vi "Rectangle Comparison.vi"(6 "Line Border":cluster{"Top":dbl, "Bottom":dbl}={"Top"=6.0, "Bottom"=1.0}, 9 "Second":dbl[](array[numeric]), 11 "First":dbl[](array[numeric])) -> (0 "Rect":T1, 1 "Line":T1, 3 "Scores":T2)   [LabVIEW 2016]
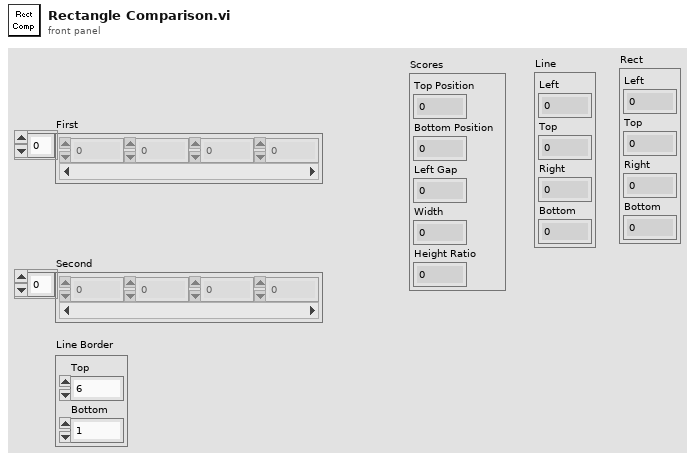
[diagram p1: front panel]
types:
  T1 = cluster{"Left":dbl, "Top":dbl, "Right":dbl, "Bottom":dbl}
  T2 = cluster{"Top Position":dbl, "Bottom Position":dbl, "Left Gap":dbl, "Width":dbl, "Height Ratio":dbl}
  T3 = cluster{"[0]":dbl, "[1]":dbl, "[2]":dbl, "[3]":dbl}
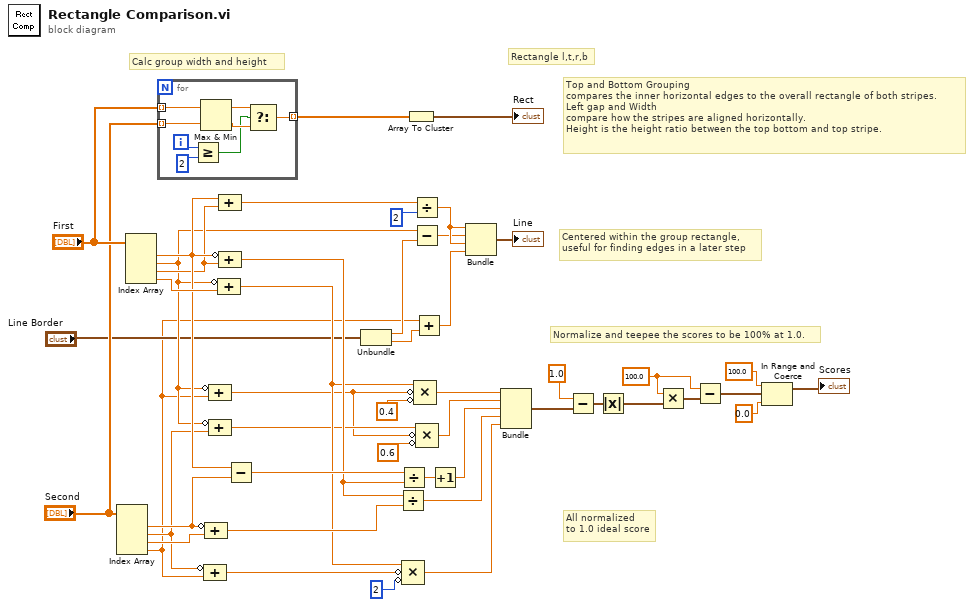
[diagram p0: block diagram]
diagram:
  w20 = 100.0 ("x/y")
  # "Centered within the group rectangle,\nuseful for finding edges in a later step"
  # "All normalized\nto 1.0 ideal score"
  # "Normalize and teepee the scores to be 100% at 1.0."
  # "Top and Bottom Grouping\ncompares the inner horizontal edges to the overall rectangle of both stripes.\nLeft gap and Width\ncompare how the stripes are aligned horizontally.\nHeight is the height ratio between the top bottom and top stripe."
  # "Calc group width and height"
  # "Rectangle l,t,r,b"
  n1 = Index Array(array="Second") -> (element #1=w44:dbl, element #2=w11:dbl, element #3=w47:dbl, element #4=w1:dbl)  [unwired: 4 in]
  n2 = Index Array(array="First") -> (element #1=w36:dbl, element #2=w10:dbl, element #3=w35:dbl, element #4=w37:dbl)  [unwired: 4 in]
  n3 = for {
    tunnel: "First" -> [w55] mode=indexing
    tunnel: "Second" -> [w54] mode=indexing
    tunnel: [w48] -> w27 mode=indexing
    i -> [w52]
    n4 = Greater Or Equal?(x=w52, y=2) -> (x >= y?=w49:bool)
    n5 = Max & Min(x=w55, y=w54) -> (max(x,y)=w51:dbl, min(x,y)=w50:dbl)
    n6 = Select(t=w51, s=w49, f=w50) -> (s? t:f=w48:dbl)
  }
  n7 = Compound Arithmetic op=ADD(invert w11, w1) -> (w45:dbl)
  n8 = Compound Arithmetic op=ADD(invert w44, w47) -> (w46:dbl)
  n9 = Compound Arithmetic op=ADD(invert w10, w1) -> (w8:dbl)
  n10 = Compound Arithmetic op=ADD(invert w10, w11) -> (w9:dbl)
  n11 = Compound Arithmetic op=ADD(invert w10, w37) -> (w12:dbl)
  n12 = Compound Arithmetic op=ADD(w36, w35) -> (w34:dbl)
  n13 = Compound Arithmetic op=ADD(invert w36, w35) -> (w42:dbl)
  n14 = Subtract(x=w36, y=w44) -> (x-y=w43:dbl)
  n15 = Unbundle("Line Border") -> ("Top"=w2:dbl, "Bottom"=w3:dbl)
  n16 = Divide(x=w42, y=w46) -> (x/y=w40:dbl)
  n17 = Divide(x=w43, y=w42) -> (x/y=w38:dbl)
  n18 = Compound Arithmetic op=MULTIPLY(w12, invert w45, invert 2) -> (w39:dbl)
  n19 = Array To Cluster(array=w27) -> (cluster=→"Rect":T3)
  n20 = Divide(x=w34, y=2) -> (x/y=w33:dbl)
  n21 = Subtract(x=w10, y=w2) -> (x-y=w31:dbl)
  n22 = Add(x=w1, y=w3) -> (x+y=w25:dbl)
  n23 = Compound Arithmetic op=MULTIPLY(w12, invert w8, invert 0.4 ("y")) -> (w41:dbl)
  n24 = Compound Arithmetic op=MULTIPLY(w9, invert w8, invert 0.6 ("y")) -> (w7:dbl)
  n25 = Increment(x=w38) -> (x+1=w24:dbl)
  n26 = Bundle(w33, w31, w33, w25) -> (→"Line":cluster{dbl, dbl, dbl, dbl})  [unwired: 1 in]
  n27 = Bundle(w41, w7, w24, w40, w39) -> (w14:cluster{dbl, dbl, dbl, dbl, dbl})  [unwired: 1 in]
  n28 = Subtract(x=1.0 ("y"), y=w14) -> (x-y=w18:cluster{dbl, dbl, dbl, dbl, dbl})
  n29 = Absolute Value(x=w18) -> (abs(x)=w21:cluster{dbl, dbl, dbl, dbl, dbl})
  n30 = Multiply(x=w20, y=w21) -> (x*y=w22:cluster{dbl, dbl, dbl, dbl, dbl})
  n31 = Subtract(x=w20, y=w22) -> (x-y=w17:cluster{dbl, dbl, dbl, dbl, dbl})
  n32 = In Range and Coerce(upper limit=100.0, x=w17, lower limit=0.0) -> (coerced(x)=→"Scores":cluster{dbl, dbl, dbl, dbl, dbl})  [unwired: 1 out]
